vi "Read Errors.vi"(11 "Pump_1AI_1DO_2DI in":refnum<class "PM_Group.lvclass">) -> (0 "UnOFF Error":refnum<class "Sig_DA.lvclass">, 1 "UnON Error":refnum<class "Sig_DA.lvclass">, 2 "OFF Error":refnum<class "Sig_DA.lvclass">, 3 "ON Error":refnum<class "Sig_DA.lvclass">)   [LabVIEW 2019, in "PM_Group.lvclass"]
uses:
  PM_Group.lvclass
  Sig_DA_class/Sig_DA.lvclass
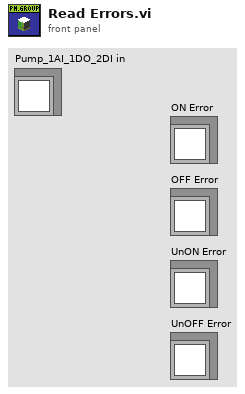
[diagram p1: front panel]
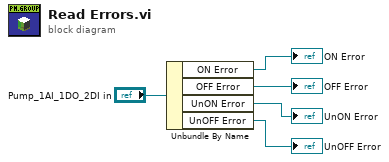
[diagram p0: block diagram]
diagram:
  n1 = Unbundle By Name("Pump_1AI_1DO_2DI in") -> ("ON Error"=→"ON Error":refnum<class "Sig_DA.lvclass">, "OFF Error"=→"OFF Error":refnum<class "Sig_DA.lvclass">, "UnON Error"=→"UnON Error":refnum<class "Sig_DA.lvclass">, "UnOFF Error"=→"UnOFF Error":refnum<class "Sig_DA.lvclass">)
